vi "from_variant.vi"(5 "LVData in":refnum<class "variant.lvclass">, 8 "error in":errorcluster, 11 "Data":variant) -> (0 "error out":errorcluster, 3 "LVData out":refnum<class "variant.lvclass">)   [LabVIEW 2020, in "variant.lvlib" / "variant.lvclass"]
uses:
  variant.lvclass
  Bytes/Bytes.lvclass/Bytes.ctl
  variant.lvclass/variant.ctl
  Type Descriptor/TD.lvclass
  DataString/DataString.lvclass
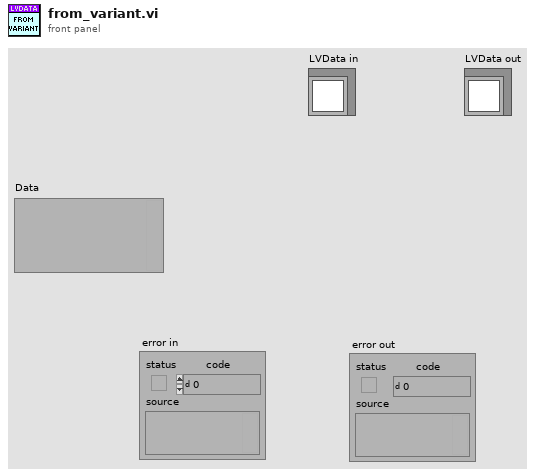
[diagram p1: front panel]
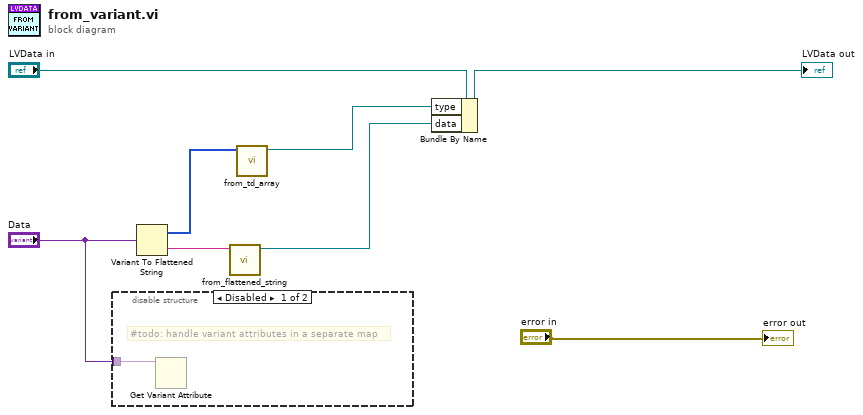
[diagram p0: block diagram]
diagram:
  n1 = disable-structure shown="Disabled" {
    disable-tunnel: "Data" -> [w9 _]
    frame Disabled {
      # "#todo: handle variant attributes in a separate map"
      n2 = Get Variant Attribute(Variant=w9) -> ()  [unwired: 3 in, 4 out]
    }
    frame Enabled {
    }
  }
  n3 = Variant To Flattened String(Variant="Data") -> (data string=w2:string, 1:w4:i16[])
  n4 = call "from_flattened_string.vi"("string_data"=w2) -> ("DataString out"=w1:refnum<class "DataString.lvclass">)  [unwired: 9 in, 1 out]
  n5 = call "from_td_array.vi"("type descriptor array"=w4) -> ("TypeDescriptor out"=w3:refnum<class "TD.lvclass">)  [unwired: 9 in, 1 out]
  n6 = Bundle By Name(cluster="LVData in", "type"=w3, "data"=w1) -> (→"LVData out":refnum<class "variant.lvclass">)
  "error out" <- "error in"
